vi "Missing.vi"() -> (2 "Missing":refnum<k24>)   [LabVIEW 2017, in "Localization.lvlib" / "Excel Support.lvlib"]
doc: "<B>Description:</B> Returns the System.Object Missing .NET class.\n\n<B>Date:</B> 11/2022\n<B>Author:</B> Luke Jarocki, Choose Movement Consulting"
uses:
  Excel Support.lvlib
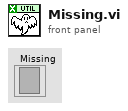
[diagram p1: front panel]
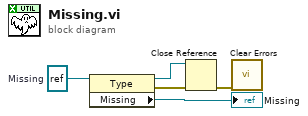
[diagram p0: block diagram]
diagram:
  w5 = refnum<k24> refnum  # Missing
  n1 = property class="Type"(reference=w5) -> (reference out=w3:refnum<k24>, error out=w2:errorcluster, "Missing"=→"Missing":refnum<k24>)  [unwired: 1 in]
  n2 = Close Reference(reference=w3, error in (no error)=w2) -> (error out=w1:errorcluster)
  n3 = call <vilib>:"Clear Errors.vi"("error in (no error)"=w1) -> ()  [unwired: 5 in, 2 out]
